vi "URAPI_ForStart_num.vi"(0 "Iterations":u16=10, 3 "URAPI Script":T1={"Script"="", "Whiles"=[], "Ifs"=[], "Supress Err"=TRUE, "Errors"=""}) -> (2 "variable":string, 5 "URAPI Script Out":T1={"Script"="", "Whiles"=[], "Ifs"=[], "Supress Err"=TRUE, "Errors"=""})   [LabVIEW 2012]
doc: "Begins the execution of a for loop. The loop will execute the specified number of \"iterations\".\nNote: requires Loop end VI."
uses:
  <userlib>/BotSpeak/VIs/Direct/URAPI_Control.ctl
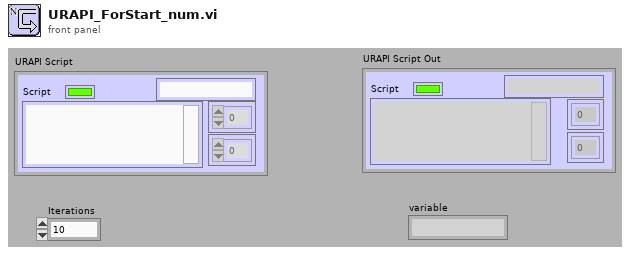
[diagram p1: front panel]
types:
  T1 = typedef "URAPI_Control.ctl" = cluster{"Script":string, "Whiles":u8[], "Ifs":u8[], "Supress Err":bool, "Errors":string}
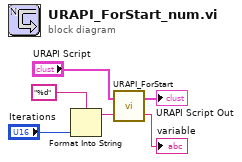
[diagram p0: block diagram]
diagram:
  n1 = Format Into String(format string="%d", "Iterations") -> (resulting string=w3:string)  [unwired: 2 in, 1 out]
  n2 = call <userlib>:"URAPI_ForStart.vi"("Iterations"=w3, "URAPI Script"="URAPI Script") -> ("variable"=→"variable":string, "URAPI Script Out"=→"URAPI Script Out":T1)  [unwired: 2 in]
